vi "LMS_StartStream.vi"(8 "error in (no error)":errorcluster, 10 "stream 2":T1) -> (0 "error out":errorcluster)   [LabVIEW 2013, in "LMS_LV_Drv.lvlib"]
uses:
  LMS_LV_Drv.lvlib
  Stream_ctl.ctl
  LimeSuite.dll
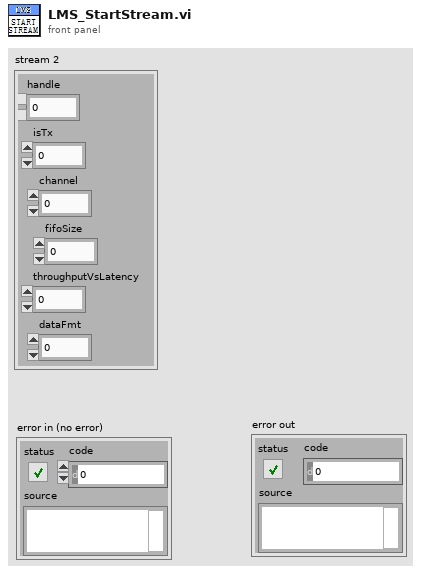
[diagram p1: front panel]
types:
  T1 = typedef "Stream_ctl.ctl" = cluster{"handle":u64, "isTx":u8, "channel":u32, "fifoSize":u32, "throughputVsLatency":dbl, "dataFmt":u32}
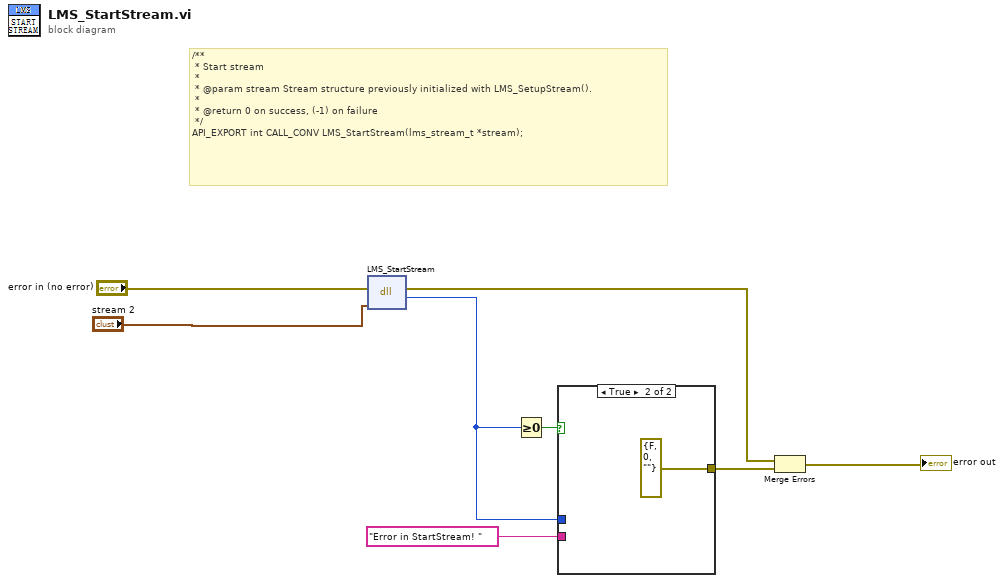
[diagram p0: block diagram]
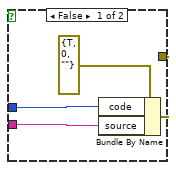
[diagram p2: hidden frame]
diagram:
  # "/**\n * Start stream\n *\n * @param stream Stream structure previously initialized with LMS_SetupStream().\n *\n * @return 0 on success, (-1) on failure\n */\nAPI_EXPORT int CALL_CONV LMS_StartStream(lms_stream_t *stream);"
  n1 = dll-call lib="PTH1mabs CUsersOTADesktop书籍出版程序8.第八章LimeSDR_LabVIEW_Driver-master\nLimeSuite.dll" fn="LMS_StartStream"(error in="error in (no error)", "steam"="stream 2") -> (error out=w2:errorcluster, "return type"=w3:i32)  [unwired: 3 in, 1 out]
  n2 = Greater Or Equal To 0?(x=w3) -> (x >= 0?=w6:bool)
  n3 = case shown="True" w6 {
    tunnel: [w11 errorcluster {"status"=FALSE, "code"=0, "source"=""} ("error in")] -> w4
    tunnel: w3 -> [w10 _]
    tunnel: "Error in StartStream! " ("source") -> [w9 _]
    frame False {
      n4 = Bundle By Name(cluster=errorcluster {"status"=TRUE, "code"=0, "source"=""} ("error in"), "code"=w10, "source"=w9) -> (w11:errorcluster)
    }
    frame True {
    }
  }
  n5 = Merge Errors(w2, w4) -> (→"error out":errorcluster)
